vi "05_dosing.vi"() -> ()   [LabVIEW 2024]
uses:
  <vilib>/Utility/error.llb/DialogType.ctl
  <vilib>/Waveform/WDTOps.llb/WDT Waveform to XY Pairs DBL.vi
  <instrlib>/Tektronix DMM40x0 Series/Tektronix DMM40x0 Series.lvlib
  <vilib>/Utility/file.llb/Write Delimited Spreadsheet (DBL).vi
panel:
  in  "OK Button":bool
  in  "error in":errorcluster
  out "Waveform Graph 2":dbl[](array[numeric])
  out "error out":errorcluster
  out "STABLE":bool
  in  "Serial Communication":T1={"Baud Rate"=9600, "Parity"=0, "Data Bits"=8, "Stop Bits"=10, "Flow Control"=0} {"Flow Control" items=["None", "XON/XOFF", "RTS/CTS", "XON/XOFF & RTS/CTS", "DTR/DSR", "XON/XOFF & DTR/DSR"]; "Stop Bits" items=["1.0"=10, "1.5"=15, "2.0"=20]; "Data Bits" items=["7"=7, "8"=8]; "Parity" items=["None", "Odd", "Even", "Mark", "Space"]; "Baud Rate" items=["300"=300, "600"=600, "1200"=1200, "2400"=2400, "4800"=4800, "9600"=9600, "19200"=19200]}
  in  "COM PORT (COM2)":refnum<visa-resource-name>
  out "Stability threshold":dbl format="%#_13g"
  out "Waveform Graph":dbl[](graph)
  # "Voltmeter Serial Configuration"
  # "DEFAULT SETTINGS:\n\nTimeout (10000 ms)\nTrigger Count (5000)\nSample Count (1)\n\n****DC VOLTAGE***"
  # "Voltmeter Stability"
  # "0 - Stability threshold not met\n1 - Stability threshold met\n\n\n\n*stability (+/-0.05 mV) of last 15 pts"
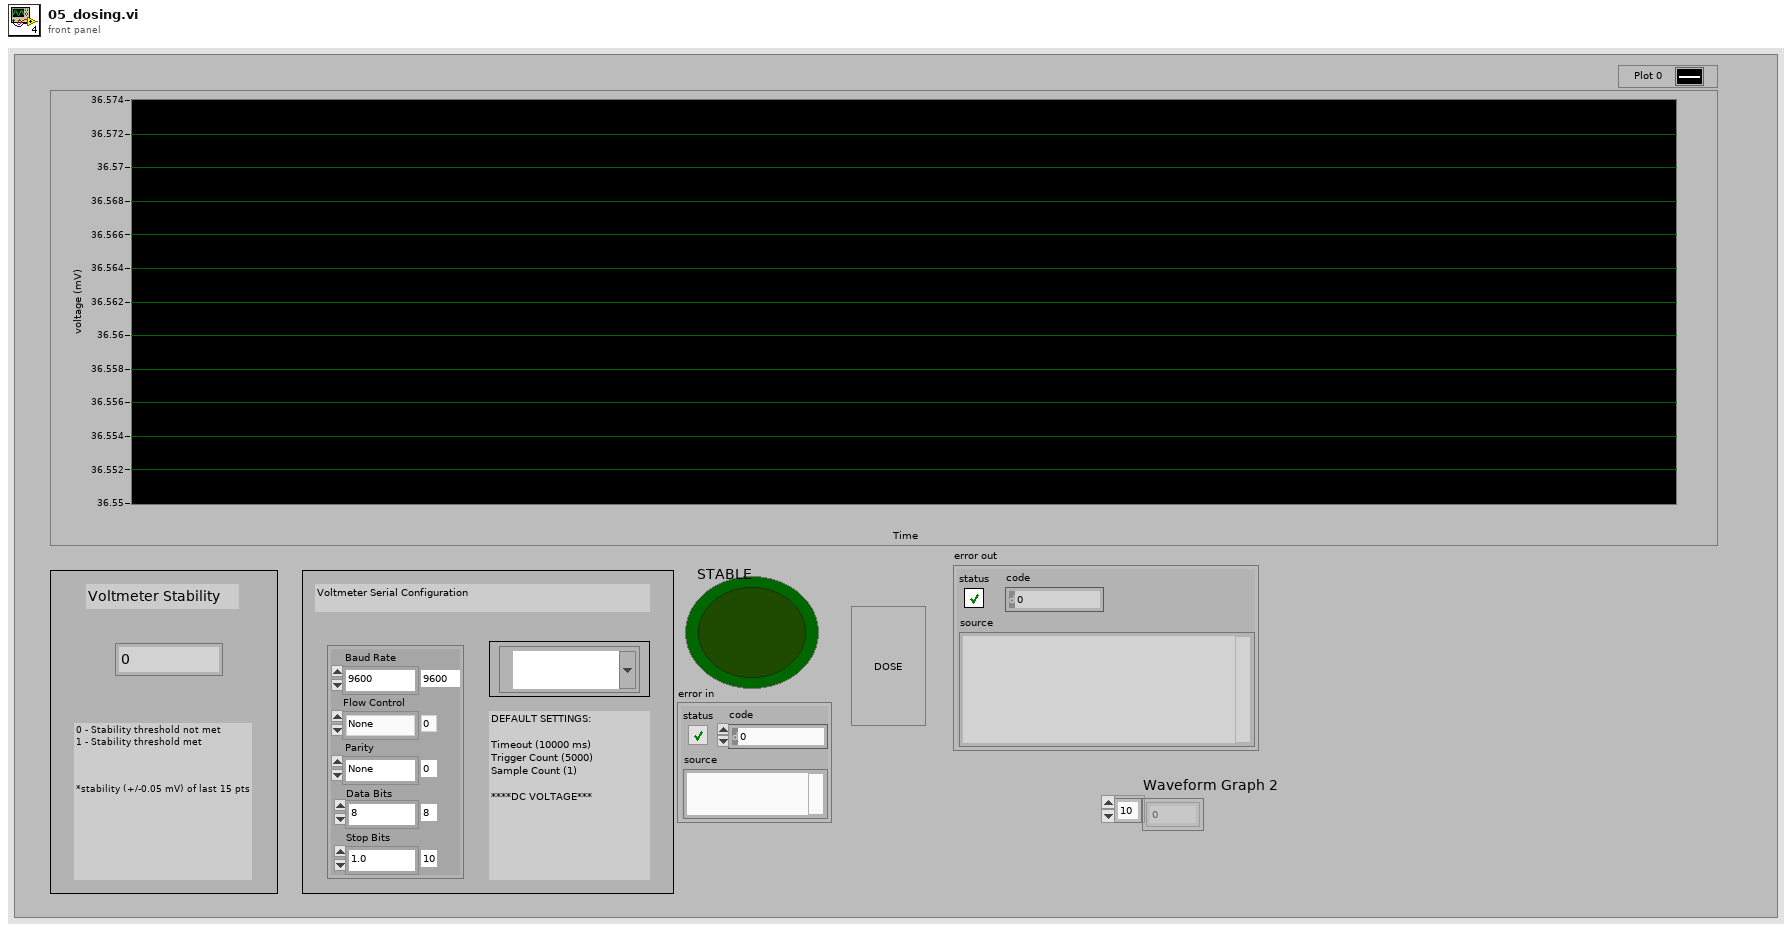
[diagram p1: front panel]
types:
  T1 = cluster{"Baud Rate":u32, "Parity":u16, "Data Bits":u16, "Stop Bits":u16, "Flow Control":u16}
  T2 = typedef "DialogType.ctl" = u16
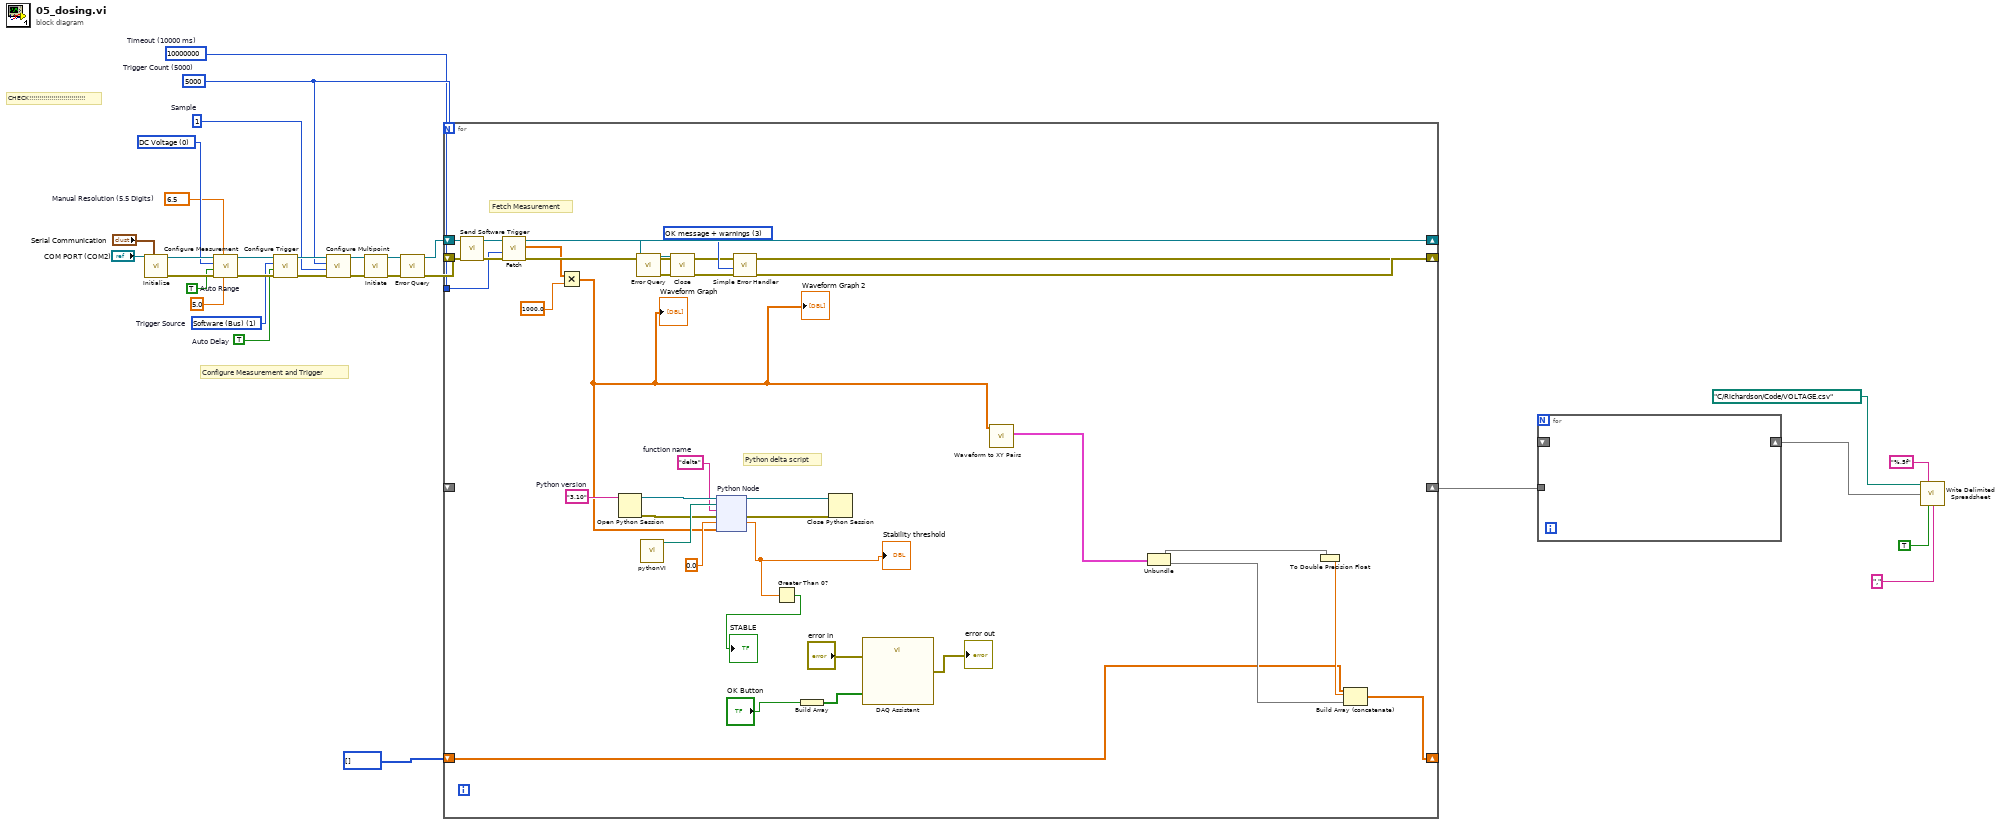
[diagram p0: block diagram]
diagram:
  w17 = u16 0 items=["DC Voltage", "AC Voltage", "2 - Wire Resistance", "4 - Wire Resistance", "DC Current", "AC Current", "Frequency", "Period", "Continuity", "Diode Checking", "Temperature", "Capacitance"] ("Function (0: DC Voltage)")
  w8 = u32 10000000  # Timeout (10000 ms)
  w9 = 1  # Sample
  w16 = 5000  # Trigger Count (5000)
  w10 = 6.5 items=["4.5"=4.5, "5.5"=5.5, "6.5"=6.5]  # Manual Resolution (5.5 Digits)
  w18 = TRUE  # Auto Delay
  w19 = u16 1 items=["Immediate", "Software (Bus)", "External"]  # Trigger Source
  w20 = TRUE  # Auto Range
  w23 = T2 3 items=["no dialog", "OK message", "continue or stop message", "OK message + warnings", "continue/stop + warnings"] ("type of dialog (OK msg:1)")
  # "CHECK!!!!!!!!!!!!!!!!!!!!!!!!!!!!"
  # "Configure Measurement and Trigger"
  n1 = call <instrlib>:"Initialize.vi"("Serial Configuration"="Serial Communication", "VISA resource name"="COM PORT (COM2)") -> ("error out"=w35:errorcluster, "VISA resource name out"=w36:refnum<visa-resource-name>)  [unwired: 3 in, 5 out]
  n2 = call <instrlib>:"Configure Measurement.vi"("Manual Range (1.0)"=5.0, "Manual Resolution (5.5 Digits)"=w10, "error in (no error)"=w35, "Auto Range (T:Enable)"=w20, "Function (0: DC Voltage)"=w17, "VISA resource name"=w36) -> ("error out"=w33:errorcluster, "VISA resource name out"=w34:refnum<visa-resource-name>)  [unwired: 4 out]
  n3 = call <instrlib>:"Configure Trigger.vi"("error in (no error)"=w33, "Auto Delay (T: Enable)"=w18, "Trigger Source (0: Immediate)"=w19, "VISA resource name"=w34) -> ("error out"=w31:errorcluster, "VISA resource name out"=w32:refnum<visa-resource-name>)  [unwired: 1 in, 5 out]
  n4 = call <instrlib>:"Configure Multipoint.vi"("error in (no error)"=w31, "Sample Count (1)"=w9, "Trigger Count (1)"=w16, "VISA resource name"=w32) -> ("error out"=w28:errorcluster, "VISA resource name out"=w29:refnum<visa-resource-name>)  [unwired: 6 out]
  n5 = call <instrlib>:"Initiate.vi"("error in (no error)"=w28, "VISA resource name"=w29) -> ("error out"=w15:errorcluster, "VISA resource name out"=w14:refnum<visa-resource-name>)  [unwired: 8 out]
  n6 = call <instrlib>:"Error Query.vi"("error in (no error)"=w15, "VISA resource name"=w14) -> ("error out"=w12:errorcluster, "VISA resource name out"=w13:refnum<visa-resource-name>)  [unwired: 8 out]
  n7 = for {
    N: w16 -> [_]
    shift-right: [w66] -> w25
    shift-left: w12 -> [w62]
    shift-right: [w67] -> w27
    shift-left: w13 -> [w63]
    tunnel: w8 -> [w61]
    shift-right: [w38] -> w2
    shift-left: _ -> [_]
    shift-right: [w37] -> _
    shift-left: i32[] [] -> [w40]
    w54 = "delta"  # function name
    w52 = "3.10"  # Python version
    # "Python delta script"
    # "Fetch Measurement"
    n8 = call <instrlib>:"Send Software Trigger.vi"("error in (no error)"=w62, "VISA resource name"=w63) -> ("error out"=w64:errorcluster, "VISA resource name out"=w65:refnum<visa-resource-name>)  [unwired: 8 out]
    n9 = call <instrlib>:"Fetch.vi"("error in (no error)"=w64, "Timeout (10000 ms)"=w61, "VISA resource name"=w65) -> ("error out"=w66:errorcluster, "Measurements"=w60:dbl[], "VISA resource name out"=w67:refnum<visa-resource-name>)  [unwired: 6 out]
    n10 = Multiply(x=w60, y=1000.0) -> (x*y=w44:dbl[])
    "Waveform Graph" <- w44
    "Waveform Graph 2" <- w44
    n11 = Open Python Session(python version=w52) -> (session out=w58:refnum<k35>, error out=w55:errorcluster)  [unwired: 2 in]
    n12 = call "pythonVI.vi"() -> ("appended path"=w59:path)  [unwired: 11 in]
    n13 = node "Python Node"(w58, w59, w54, w55, 0.0, w44) -> (w57:refnum<k35>, w56:errorcluster, w51:dbl)  [unwired: 1 in, 2 out]
    "Stability threshold" <- w51
    n14 = Greater Than 0?(x=w51) -> (x > 0?=→"STABLE":bool)
    n15 = Build Array("OK Button") -> (w49:bool[])
    n16 = Close Python Session(session in=w57, error in=w56) -> ()  [unwired: 1 out]
    n17 = call "DAQ Assistant"("data"=w49, "error in"="error in") -> ("error out"=→"error out":errorcluster)  [unwired: 16 in, 1 out]
    n18 = call-poly <vilib>:"Waveform to XY Pairs.vi"("waveform in"=w44) -> ("XY pairs"=w39:cluster{"x":timestamp, "y":dbl}[])  [unwired: 8 in, 2 out]
    n19 = Unbundle(w39) -> (w43, w42)
    n20 = To Double Precision Float(number=w43) -> (double precision float=w41:dbl)
    n21 = Build Array (concatenate)(w40, w41, w42) -> (w37:dbl[])
  }
  n22 = call <instrlib>:"Error Query.vi"("error in (no error)"=w25, "VISA resource name"=w27) -> ("error out"=w24:errorcluster, "VISA resource name out"=w26:refnum<visa-resource-name>)  [unwired: 8 out]
  n23 = call <instrlib>:"Close.vi"("error in (no error)"=w24, "VISA resource name"=w26) -> ("error out"=w30:errorcluster)  [unwired: 9 out]
  n24 = call <vilib>:"Simple Error Handler.vi"("type of dialog (OK msg:1)"=w23, "error in (no error)"=w30) -> ()  [unwired: 8 out]
  n25 = for {
    shift-right: [_] -> w7
    shift-left: _ -> [_]
    tunnel: w2 -> [_]
  }
  n26 = call-poly <vilib>:"Write Delimited Spreadsheet.vi"("file path (dialog if empty)"=path "C:/Richardson/Code/VOLTAGE.csv", "format (%.3f)"="%.5f", "1D data"=w7, "transpose? (no:F)"=TRUE, "delimiter (\\t)"="," ("delimiter (\\t)")) -> ()  [unwired: 9 in, 2 out]
